vi "SE_E5_P8.vi"() -> ()   [LabVIEW 2015]
panel:
  in  "Cámara OFF":bool
  in  "Cámara ON":bool
  out "Estado":bool
  in  "Pedo":bool
  in  "Sobrio":bool
  in  "Puerta OFF":bool
  out "Camaras":bool
  out "Puerta":bool
  in  "Puerta ON":bool
  in  "stop":bool
  out "Ventilador":bool
  out "Bomba":bool
  in  "Ventilador OFF":bool
  in  "Ventilador ON":bool
  in  "Bomba OFF":bool
  in  "Bomba ON":bool
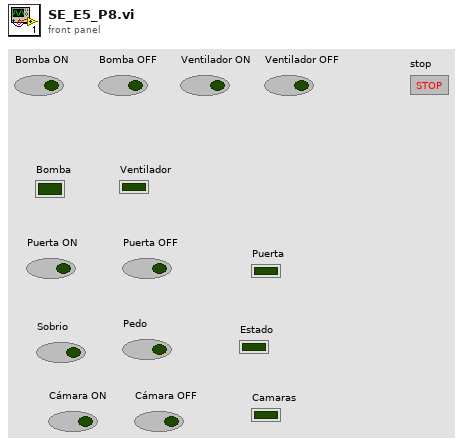
[diagram p1: front panel]
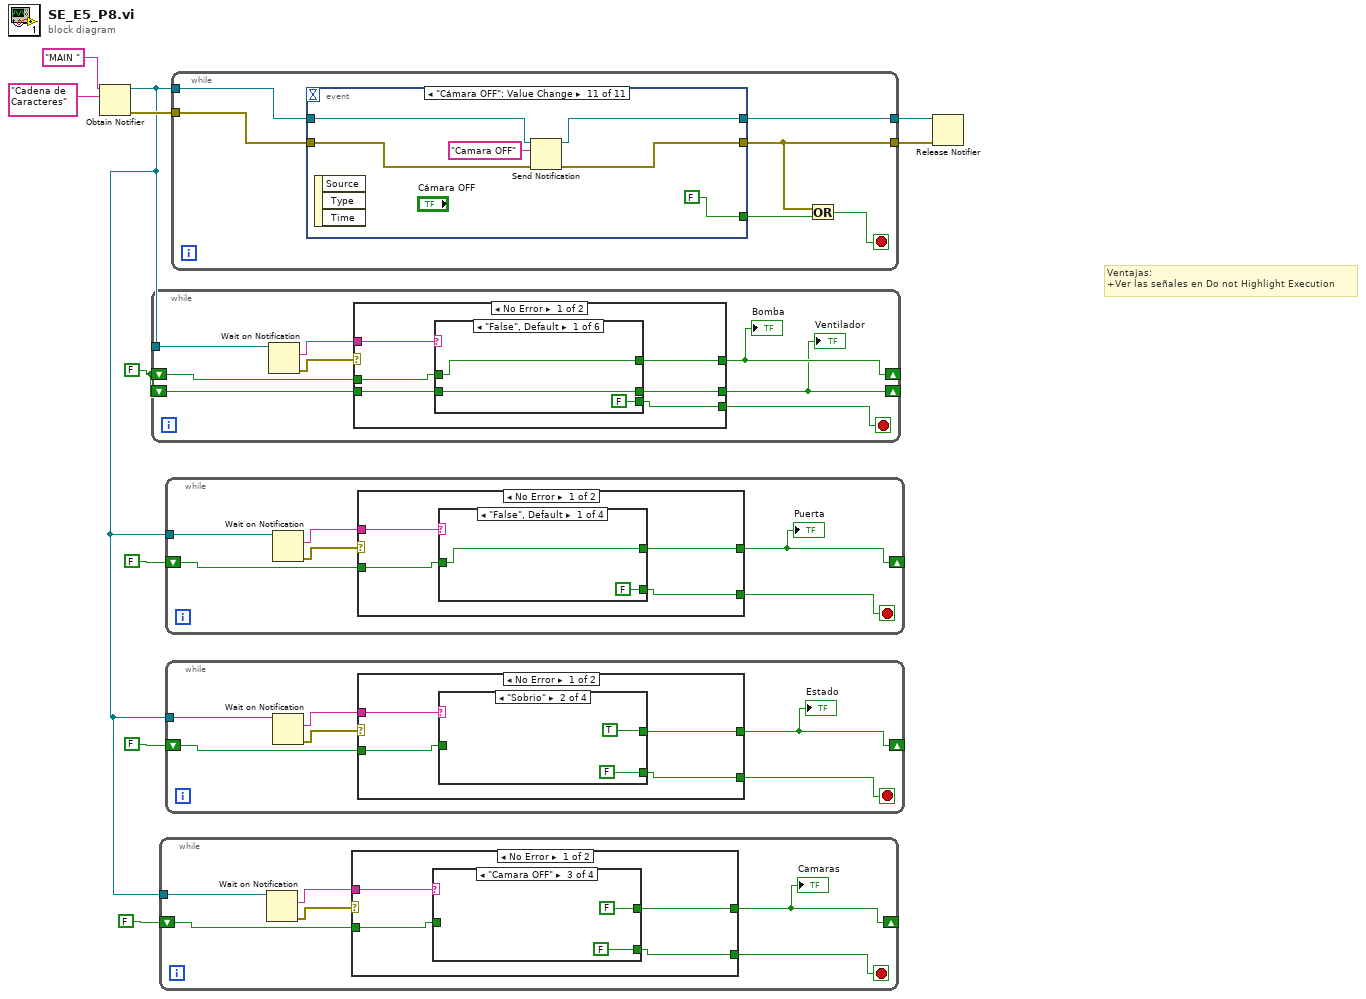
[diagram p0: block diagram]
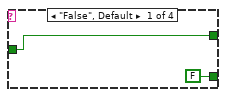
[diagram p2: hidden frame]
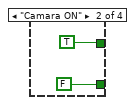
[diagram p3: hidden frame]
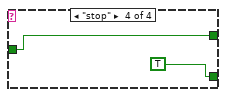
[diagram p4: hidden frame]
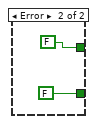
[diagram p5: hidden frame]
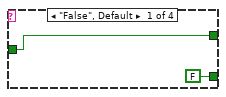
[diagram p6: hidden frame]
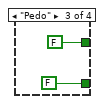
[diagram p7: hidden frame]
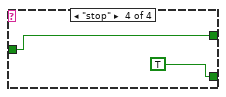
[diagram p8: hidden frame]
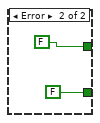
[diagram p9: hidden frame]
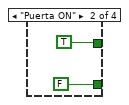
[diagram p10: hidden frame]
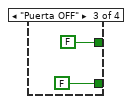
[diagram p11: hidden frame]
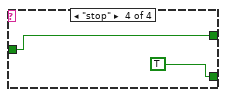
[diagram p12: hidden frame]
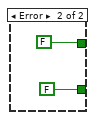
[diagram p13: hidden frame]
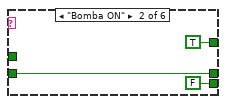
[diagram p14: hidden frame]
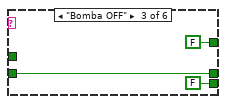
[diagram p15: hidden frame]
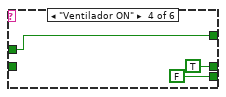
[diagram p16: hidden frame]
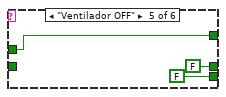
[diagram p17: hidden frame]
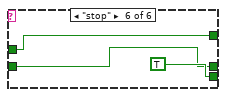
[diagram p18: hidden frame]
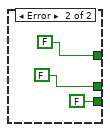
[diagram p19: hidden frame]
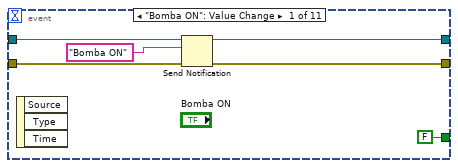
[diagram p20: hidden frame]
diagram:
  w5 = FALSE
  # "Ventajas:\n+Ver las señales en Do not Highlight Execution"
  n1 = Obtain Notifier(name (unnamed)="MAIN ", notification data type="Cadena de Caracteres") -> (notifier out=w1:refnum<notifier>, error out=w8:errorcluster)  [unwired: 2 in, 1 out]
  n2 = while {
    tunnel: w1 -> [w18]
    shift-right: [w12] -> _
    shift-left: w5 -> [w15]
    shift-right: [w11] -> _
    shift-left: w5 -> [w14]
    stop <- w13 stop-if-true
    n3 = Wait on Notification(notifier=w18) -> (notification=w16:string, error out=w17:errorcluster)  [unwired: 3 in, 2 out]
    n4 = case shown="No Error" w17 {
      tunnel: w16 -> [w24 _]
      tunnel: w15 -> [w23 _]
      tunnel: w14 -> [w22 _]
      tunnel: [w21 FALSE] -> w12
      tunnel: [w20 FALSE] -> w11
      tunnel: [w19 FALSE] -> w13
      frame No Error {
        n5 = case shown="\"False\", Default" w24 {
          tunnel: w23 -> [w27 _ _ w36 w37 w41]
          tunnel: w22 -> [w26 w29 w32 _ _ w40]
          tunnel: [w27 TRUE FALSE w36 w37 w41] -> w21
          tunnel: [w26 w29 w32 TRUE FALSE w40] -> w20
          tunnel: [FALSE FALSE FALSE FALSE FALSE TRUE] -> w19
          frame "False", Default {
          }
          frame "Bomba ON" {
          }
          frame "Bomba OFF" {
          }
          frame "Ventilador ON" {
          }
          frame "Ventilador OFF" {
          }
          frame "stop" {
          }
        }
      }
      frame Error {
      }
    }
    "Bomba" <- w12
    "Ventilador" <- w11
  }
  n6 = while {
    tunnel: w1 -> [w51]
    shift-right: [w46] -> _
    shift-left: FALSE -> [w48]
    stop <- w47 stop-if-true
    n7 = Wait on Notification(notifier=w51) -> (notification=w49:string, error out=w50:errorcluster)  [unwired: 3 in, 2 out]
    n8 = case shown="No Error" w50 {
      tunnel: w49 -> [w55 _]
      tunnel: w48 -> [w54 _]
      tunnel: [w53 FALSE] -> w46
      tunnel: [w52 FALSE] -> w47
      frame No Error {
        n9 = case shown="\"Camara OFF\"" w55 {
          tunnel: w54 -> [w57 _ _ w62]
          tunnel: [w57 TRUE FALSE w62] -> w53
          tunnel: [FALSE FALSE FALSE TRUE] -> w52
          frame "False", Default {
          }
          frame "Camara ON" {
          }
          frame "Camara OFF" {
          }
          frame "stop" {
          }
        }
      }
      frame Error {
      }
    }
    "Camaras" <- w46
  }
  n10 = while {
    tunnel: w1 -> [w71]
    shift-right: [w66] -> _
    shift-left: FALSE -> [w68]
    stop <- w67 stop-if-true
    n11 = Wait on Notification(notifier=w71) -> (notification=w69:string, error out=w70:errorcluster)  [unwired: 3 in, 2 out]
    n12 = case shown="No Error" w70 {
      tunnel: w69 -> [w75 _]
      tunnel: w68 -> [w74 _]
      tunnel: [w73 FALSE] -> w66
      tunnel: [w72 FALSE] -> w67
      frame No Error {
        n13 = case shown="\"False\", Default" w75 {
          tunnel: w74 -> [w77 _ _ w82]
          tunnel: [w77 TRUE FALSE w82] -> w73
          tunnel: [FALSE FALSE FALSE TRUE] -> w72
          frame "False", Default {
          }
          frame "Puerta ON" {
          }
          frame "Puerta OFF" {
          }
          frame "stop" {
          }
        }
      }
      frame Error {
      }
    }
    "Puerta" <- w66
  }
  n14 = while {
    tunnel: w1 -> [w91]
    shift-right: [w86] -> _
    shift-left: FALSE -> [w88]
    stop <- w87 stop-if-true
    n15 = Wait on Notification(notifier=w91) -> (notification=w89:string, error out=w90:errorcluster)  [unwired: 3 in, 2 out]
    n16 = case shown="No Error" w90 {
      tunnel: w89 -> [w95 _]
      tunnel: w88 -> [w94 _]
      tunnel: [w93 FALSE] -> w86
      tunnel: [w92 FALSE] -> w87
      frame No Error {
        n17 = case shown="\"Sobrio\"" w95 {
          tunnel: w94 -> [w97 _ _ w102]
          tunnel: [w97 TRUE FALSE w102] -> w93
          tunnel: [FALSE FALSE FALSE TRUE] -> w92
          frame "False", Default {
          }
          frame "Sobrio" {
          }
          frame "Pedo" {
          }
          frame "stop" {
          }
        }
      }
      frame Error {
      }
    }
    "Estado" <- w86
  }
  n18 = while {
    tunnel: w1 -> [w111]
    tunnel: w8 -> [w110]
    tunnel: [w108] -> w6
    tunnel: [w109] -> w7
    stop <- w107 stop-if-true
    n19 = event shown="[10] \"Cámara OFF\": Value Change" {
      selector: _ -> [_ _ _ _ _ _ _ _ _ _ _]
      dyn-events: _ -> [_ _ _ _ _ _ _ _ _ _ _]
      timeout: _ -> [_ _ _ _ _ _ _ _ _ _ _]
      tunnel: w111 -> [w117 w121 w126 w133 w140 w146 w151 w155 w161 w167 w172]
      tunnel: w110 -> [w116 w120 w125 w132 w139 w145 w150 w154 w160 w166 w171]
      tunnel: [w114 w122 w128 w134 w137 w144 w149 w156 w162 w168 w174] -> w108
      tunnel: [w113 w123 w129 w135 w138 w147 w148 w157 w163 w169 w175] -> w109
      tunnel: [FALSE FALSE FALSE FALSE TRUE FALSE _ FALSE FALSE FALSE FALSE] -> w106
      event "Bomba ON": Value Change {
        n20 = event-data() -> ()  [unwired: 1 in, 3 out]
        n21 = Send Notification(notification="Bomba ON", notifier=w117, error in (no error)=w116) -> (notifier out=w113:refnum<notifier>, error out=w114:errorcluster)
      }
      event "Bomba OFF": Value Change {
        n22 = event-data() -> ()  [unwired: 1 in, 3 out]
        n23 = Send Notification(notification="Bomba OFF", notifier=w121, error in (no error)=w120) -> (notifier out=w123:refnum<notifier>, error out=w122:errorcluster)
      }
      event "Ventilador ON": Value Change {
        n24 = event-data() -> ()  [unwired: 1 in, 3 out]
        n25 = Send Notification(notification="Ventilador ON", notifier=w126, error in (no error)=w125) -> (notifier out=w129:refnum<notifier>, error out=w128:errorcluster)
      }
      event "Ventilador OFF": Value Change {
        n26 = event-data() -> ()  [unwired: 1 in, 3 out]
        n27 = Send Notification(notification="Ventilador OFF", notifier=w133, error in (no error)=w132) -> (notifier out=w135:refnum<notifier>, error out=w134:errorcluster)
      }
      event "stop": Value Change {
        n28 = event-data() -> ()  [unwired: 1 in, 3 out]
        n29 = Send Notification(notification="Stop", notifier=w140, error in (no error)=w139) -> (notifier out=w138:refnum<notifier>, error out=w137:errorcluster)
      }
      event "Puerta ON": Value Change {
        n30 = event-data() -> ()  [unwired: 1 in, 3 out]
        n31 = Send Notification(notification="Puerta ON", notifier=w146, error in (no error)=w145) -> (notifier out=w147:refnum<notifier>, error out=w144:errorcluster)
      }
      event "Puerta OFF": Value Change {
        (unwired) FALSE
        n32 = event-data() -> ()  [unwired: 1 in, 3 out]
        n33 = Send Notification(notification="Puerta OFF", notifier=w151, error in (no error)=w150) -> (notifier out=w148:refnum<notifier>, error out=w149:errorcluster)
      }
      event "Sobrio": Value Change {
        n34 = event-data() -> ()  [unwired: 1 in, 3 out]
        n35 = Send Notification(notification="Sobrio", notifier=w155, error in (no error)=w154) -> (notifier out=w157:refnum<notifier>, error out=w156:errorcluster)
      }
      event "Pedo": Value Change {
        n36 = event-data() -> ()  [unwired: 1 in, 3 out]
        n37 = Send Notification(notification="Pedo", notifier=w161, error in (no error)=w160) -> (notifier out=w163:refnum<notifier>, error out=w162:errorcluster)
      }
      event "Cámara ON": Value Change {
        n38 = event-data() -> ()  [unwired: 1 in, 3 out]
        n39 = Send Notification(notification="Camara ON", notifier=w167, error in (no error)=w166) -> (notifier out=w169:refnum<notifier>, error out=w168:errorcluster)
      }
      event "Cámara OFF": Value Change {
        n40 = event-data() -> ()  [unwired: 1 in, 3 out]
        n41 = Send Notification(notification="Camara OFF", notifier=w172, error in (no error)=w171) -> (notifier out=w175:refnum<notifier>, error out=w174:errorcluster)
      }
    }
    n42 = Or(x=w108, y=w106) -> (x .or. y?=w107:bool)
  }
  n43 = Release Notifier(notifier=w7, error in (no error)=w6) -> ()  [unwired: 1 in, 3 out]
